vi "CheckStopAndReset.vi"(0 "ExperimentStopped?":refnum<vi>, 1 "MasterStop":refnum<vi>, 2 "MasterPause":refnum<vi>) -> ()   [LabVIEW 2019]
panel:
  in  "MasterPause":bool
  out "ExperimentStopped?":bool
  in  "MasterStop":bool
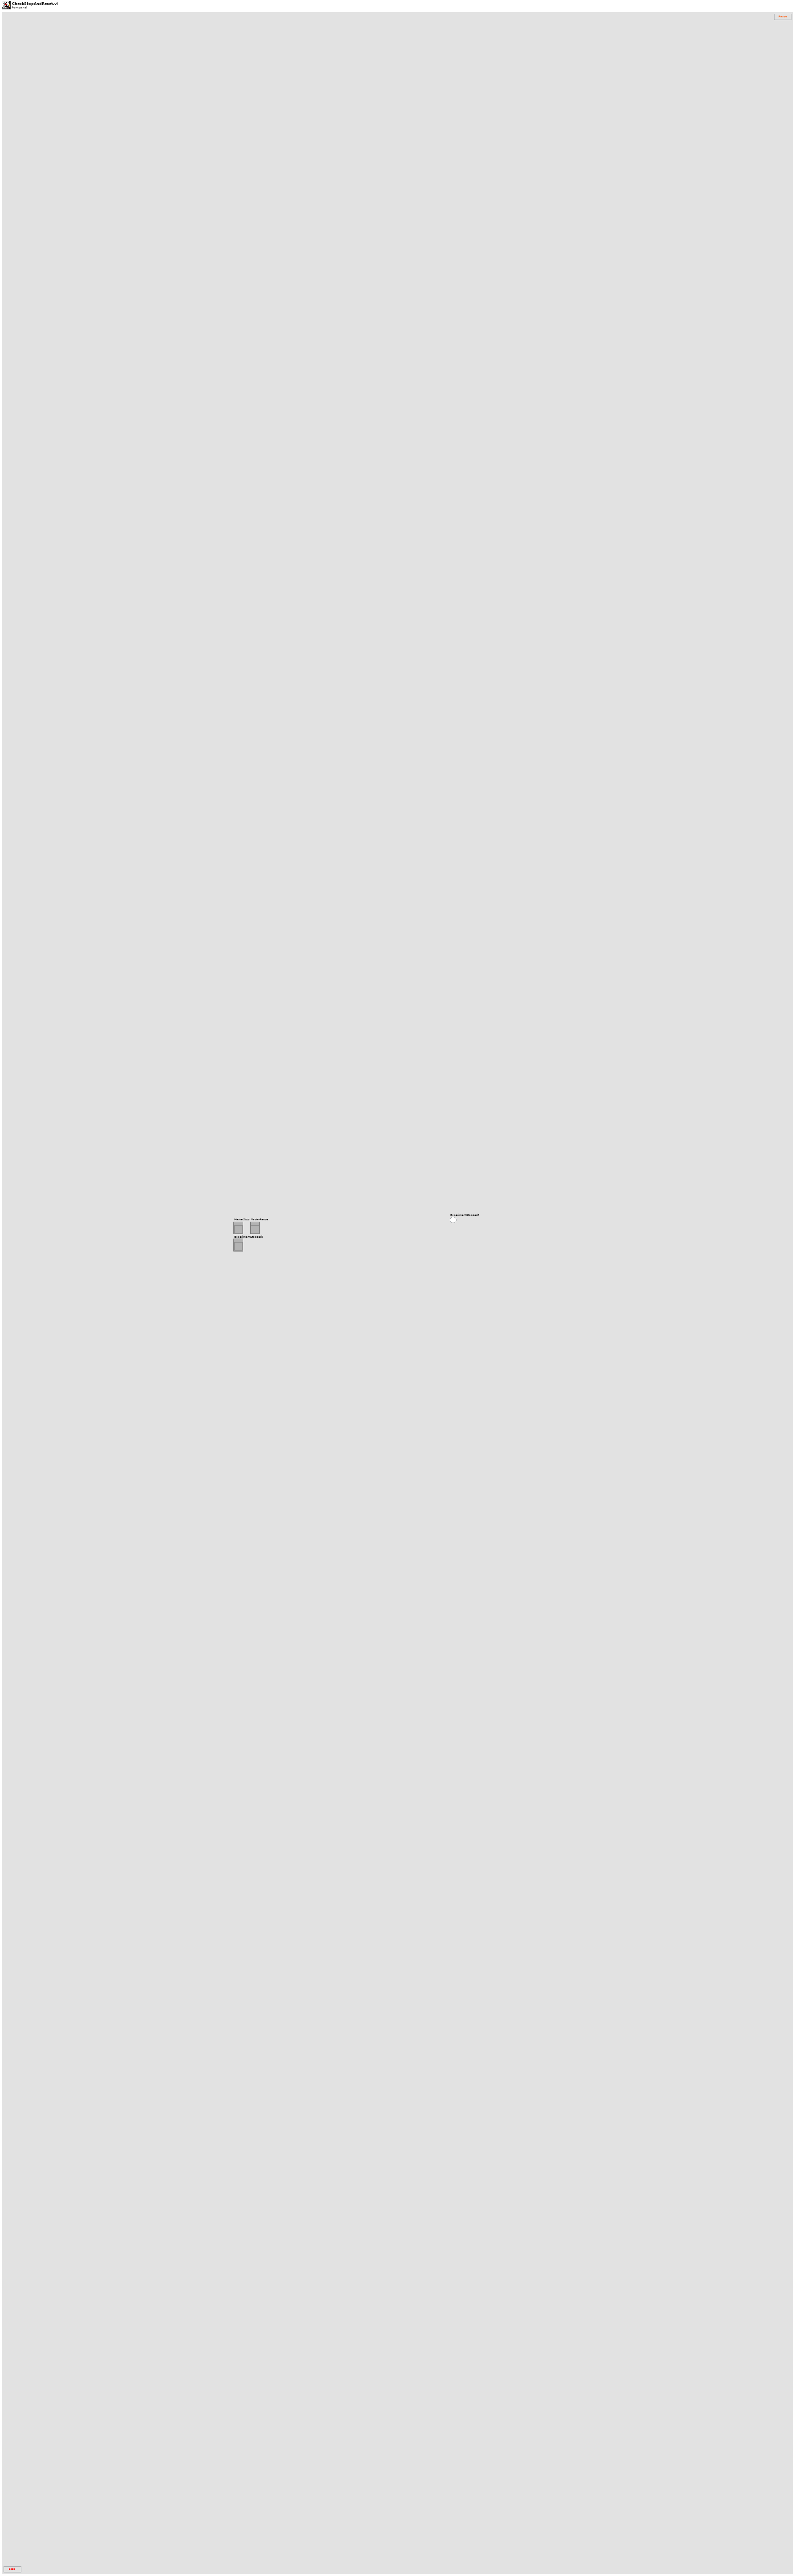
[diagram p1: front panel]
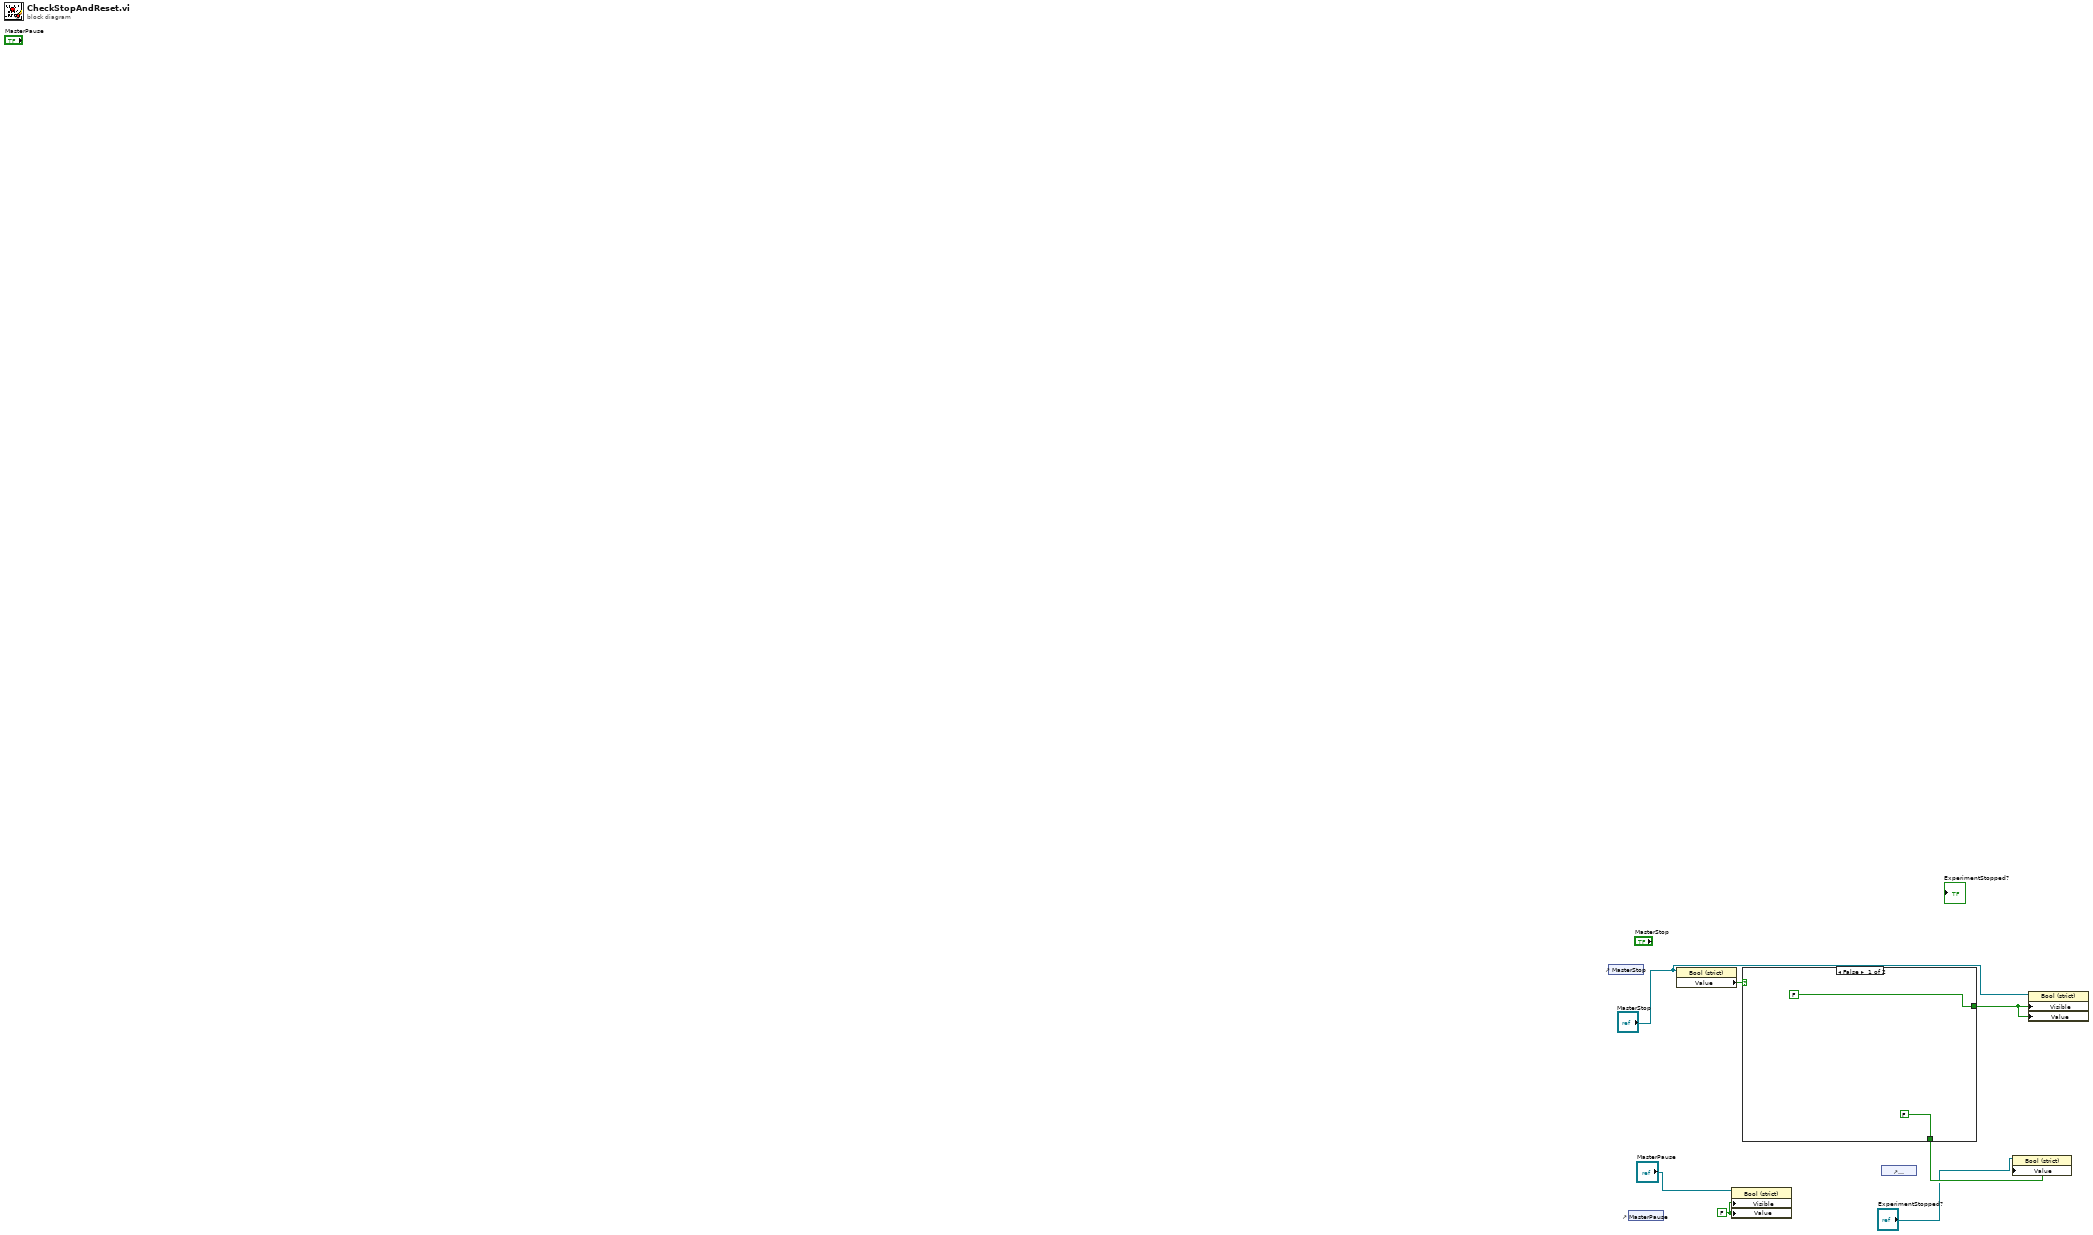
[diagram p0: block diagram]
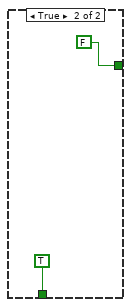
[diagram p2: hidden frame]
diagram:
  w2 = FALSE ("Value")
  n1 = control-ref of="MasterStop"() -> ()  [unwired: 1 out]
  n2 = control-ref of="MasterPause"() -> ()  [unwired: 1 out]
  n3 = property class="Bool (strict)"(reference="MasterStop") -> ("Value"=w7:bool)  [unwired: 1 in, 2 out]
  n4 = property class="Bool (strict)"(reference="MasterPause", "Visible"=w2, "Value"=w2) -> ()  [unwired: 1 in, 2 out]
  n5 = case shown="False" w7 {
    tunnel: [FALSE ("Visible") FALSE ("Visible")] -> w6
    tunnel: [FALSE TRUE] -> w5
    frame False {
    }
    frame True {
    }
  }
  n6 = control-ref of="ExperimentStopped?"() -> ()  [unwired: 1 out]
  n7 = property class="Bool (strict)"(reference="ExperimentStopped?", "Value"=w5) -> ()  [unwired: 1 in, 2 out]
  n8 = property class="Bool (strict)"(reference="MasterStop", "Visible"=w6, "Value"=w6) -> ()  [unwired: 1 in, 2 out]
